vi "Setpositionwait.vi"(7 "Tolerance[µm]":dbl format="%#_13g", 8 "error in":errorcluster, 11 "Position[µm]":dbl format="%#_13g") -> (0 "error out":errorcluster)   [LabVIEW 2014]
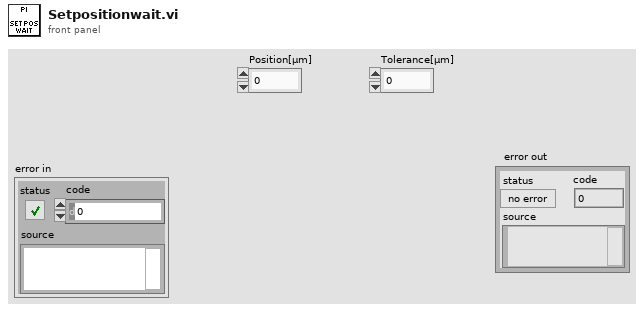
[diagram p1: front panel]
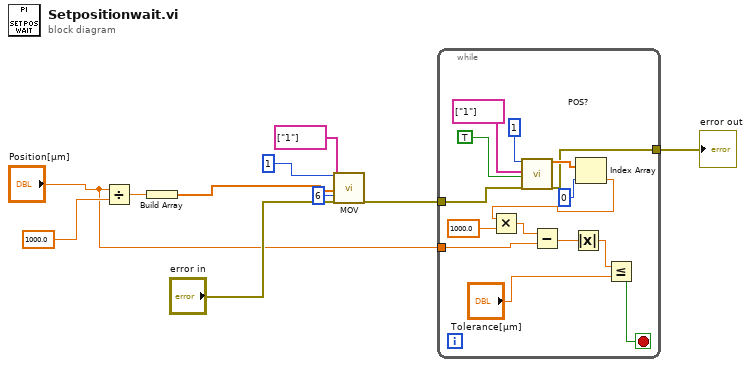
[diagram p0: block diagram]
diagram:
  n1 = Divide(x="Position[µm]", y=1000.0) -> (x/y=w5:dbl)
  n2 = Build Array(w5) -> (w7:dbl[])
  n3 = call "MOV.vi"("System no."=1, "Axes to move"=string[] ["1"], "Position values"=w7, "No.of digits"=i16 6, "error in"="error in") -> ("error out"=w3:errorcluster)  [unwired: 14 out]
  n4 = while {
    tunnel: w3 -> [w22]
    tunnel: "Position[µm]" -> [w21]
    tunnel: [w16] -> w1
    stop <- w17 stop-if-true
    n5 = call "POS?.vi"("System no."=1, "Axes to query"=string[] ["1"], "All axes?"=TRUE, "error in"=w22) -> ("Position"=w20:dbl[], "error out"=w16:errorcluster)  [unwired: 1 in, 13 out]
    n6 = Index Array(array=w20, index=0) -> (element=w15:dbl)
    n7 = Multiply(x=w15, y=1000.0) -> (x*y=w13:dbl)
    n8 = Subtract(x=w13, y=w21) -> (x-y=w12:dbl)
    n9 = Absolute Value(x=w12) -> (abs(x)=w11:dbl)
    n10 = Less Or Equal?(x=w11, y="Tolerance[µm]") -> (x <= y?=w17:bool)
  }
  "error out" <- w1
